vi "Launch Help.vi"(4 "error in":errorcluster, 6 "CHM or HLP filename (lvdialog.chm)":string="lvdialog.chm", 7 "HTML filename":string) -> (0 "error out":errorcluster)   [LabVIEW 2020, in "NI_TDMS File Viewer.lvlib"]
uses:
  <vilib>/Utility/TDMS File Viewer/NI_TDMS File Viewer.lvlib
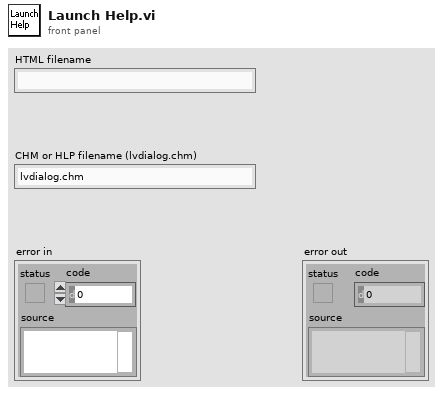
[diagram p1: front panel]
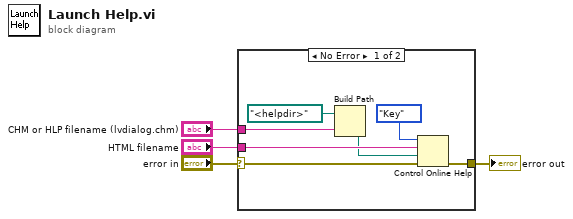
[diagram p0: block diagram]
diagram:
  n1 = case shown="No Error" "error in" {
    selector: "error in" -> [w11 w12]
    tunnel: "HTML filename" -> [w8 _]
    tunnel: "CHM or HLP filename (lvdialog.chm)" -> [w6 _]
    tunnel: [w10 w12] -> w4
    frame No Error {
      n2 = Build Path(base path=path "<helpdir>", name or relative path=w6) -> (appended path=w5:path)
      n3 = Control Online Help(1:w11, 2:w5, 3:w8, 4:enum16{"Contents", "Key", "Close"}."Key" ("Operation")) -> (0:w10:errorcluster)
    }
    frame Error {
    }
  }
  "error out" <- w4
